vi "30-20-10-2.vi"() -> ()   [LabVIEW 2025]
uses:
  <vilib>/Platform/TimedLoop/XDataNode/timing_clust.ctl
  <vilib>/Platform/TimedLoop/XDataNode/nitl_modes.ctl
  <vilib>/Platform/TimedLoop/XDataNode/wakeup.ctl
  <vilib>/rvi/Emulation/niFpgaSctlEmulationGetInTimedLoop.vi
  <vilib>/rvi/Emulation/niFpgaEmulationReportErrorSimple.vi
  <vilib>/rvi/Emulation/niFpgaGetClockAttributes.vi
  <vilib>/rvi/Emulation/niFpgaCriticalErrorInLSC.vi
  <vilib>/rvi/linearAlgebra/MatrixMultiply/simVIs/SubVI/nifxpla_MatrixMultiply_SimMatrixSizes.vi
  <vilib>/rvi/linearAlgebra/MatrixMultiply/simVIs/SubVI/nifxpla_MatrixMultiply_Sim4WireAdapterVector.vi
  <vilib>/rvi/linearAlgebra/MatrixMultiply/simVIs/SubVI/nifxpla_MatrixMultiply_SimFrameHandShake.vi
  <vilib>/rvi/linearAlgebra/MatrixMultiply/simVIs/SubVI/nifxpla_MatrixMultiply_SimEndlessCounter.vi
  <vilib>/rvi/linearAlgebra/MatrixMultiply/simVIs/SubVI/nifxpla_MatrixMultiply_SimVectorDataBuffer.vi
  <vilib>/rvi/ClientSDK/Core/DevComputerLib/Private/Multiply(dfxp64).vi
  <vilib>/rvi/ClientSDK/Core/DevComputerLib/Private/Dfxp128ToDfxp256.vi
  <vilib>/rvi/ClientSDK/Core/DevComputerLib/Private/Add(dfxp256).vi
  <vilib>/rvi/ClientSDK/Core/DevComputerLib/Private/Subtract(dfxp256).vi
  <vilib>/rvi/ClientSDK/Core/DevComputerLib/Private/ToDfxp64(dfxp256).vi
  <vilib>/platform/TimedLoop/XDataNode/XDataNode.xnode
  <vilib>/rvi/linearAlgebra/MatrixMultiply/XNode/nifxpla_MatrixMultiply.xnode
  <vilib>/rvi/linearAlgebra/MatrixMultiply/simVIs/nifxpla_MatrixMultiply_SimTemplateEinEout.vi
  <vilib>/rvi/linearAlgebra/MatrixMultiply/simVIs/nifxpla_MatrixMultiply_SimTemplateEinVout.vi
  <vilib>/rvi/linearAlgebra/MatrixMultiply/simVIs/nifxpla_MatrixMultiply_SimTemplateVinEout.vi
  <vilib>/rvi/linearAlgebra/MatrixMultiply/simVIs/nifxpla_MatrixMultiply_SimTemplateVinVout.vi
  <vilib>/Platform/TimedLoop/XDataNode/XDNodeRunTimeDep.lvlib
panel:
  out "Latency":u32
  out "Cycle Count 3":i32
  out "C3":fxp<+/-,32,16>[](array[numeric])
  out "C3+B":fxp<+/-,33,17>[](array[numeric])
  out "Cycle Count 2":i32
  out "C2":fxp<+/-,32,16>[](array[numeric])
  out "C2+B":fxp<+/-,33,17>[](array[numeric])
  out "Cycle Count":i32
  out "C1":fxp<+/-,32,16>[](array[numeric])
  out "C1+B":fxp<+/-,33,17>[](array[numeric])
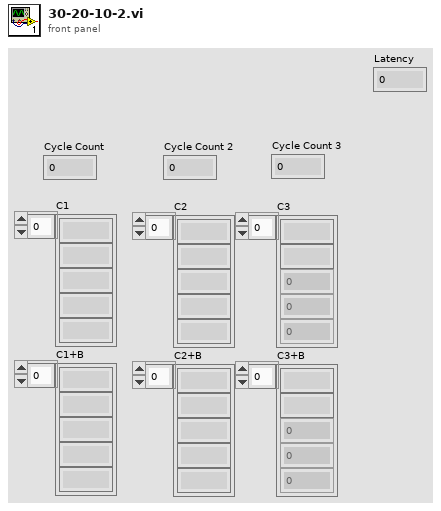
[diagram p1: front panel]
types:
  T1 = typedef "XDNodeRunTimeDep.lvlib/timing_clust.ctl" = cluster{"Expected End [f-1]":u64, "Actual End [f-1]":u64, "Finished Late? [f-1]":bool, "Expected End [i-1]":u64, "Actual End [i-1]":u64, "Finished Late? [i-1]":bool, "Expected Start [i]":u64, "Actual Start [i]":u64, "Expected Start [f]":u64, "Actual Start [f]":u64, "Source Name":string, "Structure Name":string, "Period":i64, "Deadline":i64, "Offset":i64, "Start":i64, "Priority":i32, "Timeout":i32, "Mode":T2, "Wakeup Reason":T3, "Error":errorcluster, "Source Type":string, "Secondary Source Type":string, "Global End Time":u64, "Global Start Time":u64, "Frame Duration":u64, "Iteration Duration":u64, "Assigned CPU":i32, "I/O Scan Engine Mode":u32}
  T2 = typedef "XDNodeRunTimeDep.lvlib/nitl_modes.ctl" = enum32{"No Change", "Process missed periods, maintain original phase", "Discard missed periods, maintain original phase", "Process missed periods, ignore original phase", "Discard missed periods, ignore original phase"}
  T3 = typedef "XDNodeRunTimeDep.lvlib/wakeup.ctl" = enum32{"Normal", "Aborted", "Asynchronous wakeup", "Timing source error", "Timed loop error", "Timeout"}
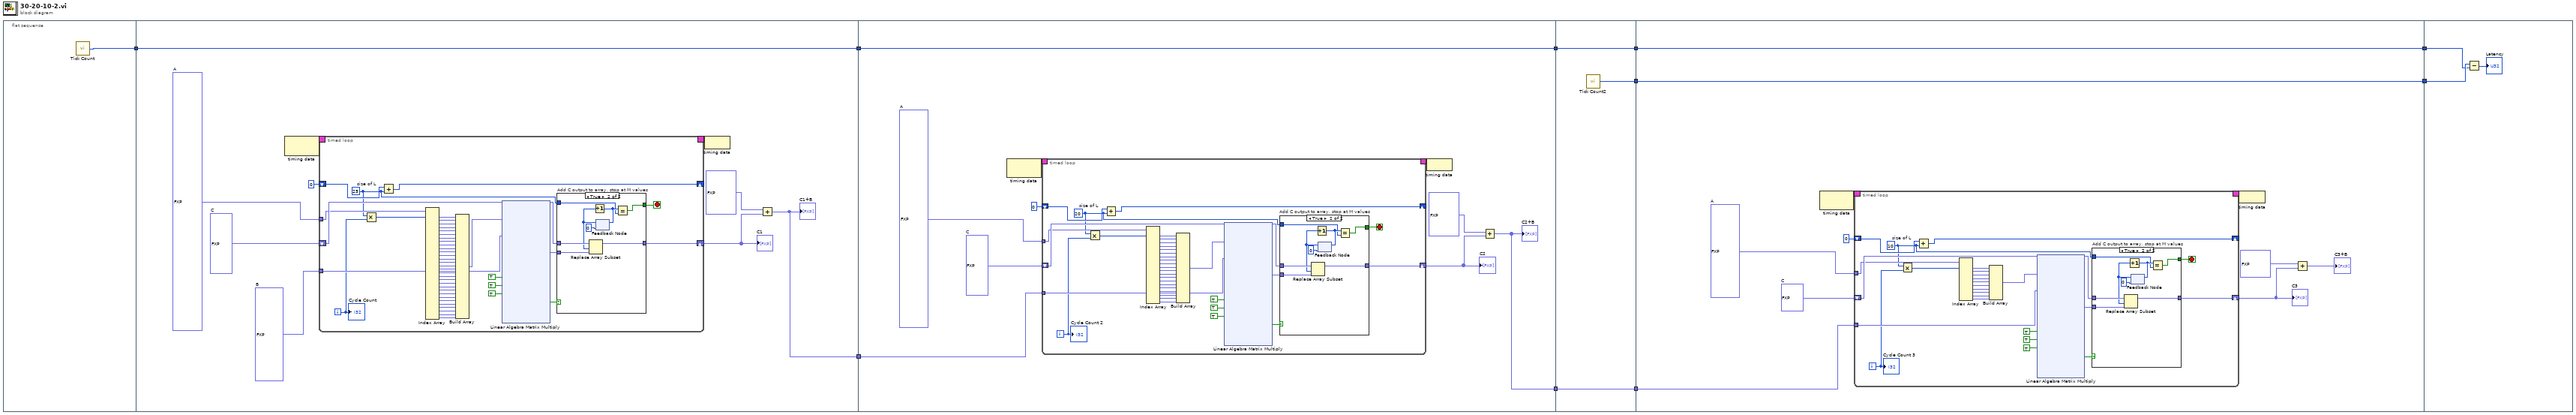
[diagram p0: block diagram]
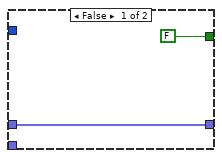
[diagram p2: hidden frame]
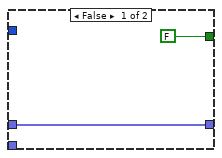
[diagram p3: hidden frame]
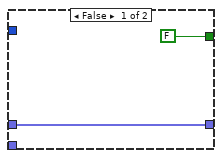
[diagram p4: hidden frame]
diagram:
  n1 = flat-sequence {
    tunnel: [w11] -> w10
    tunnel: [w13] -> w9
    tunnel: [w12] -> w8
    tunnel: w10 -> [w12]
    tunnel: w9 -> [w84]
    tunnel: [w83] -> w7
    tunnel: w8 -> [w82]
    tunnel: [w82] -> w6
    tunnel: w7 -> [w144]
    tunnel: [w144] -> w5
    tunnel: w6 -> [w143]
    tunnel: [w143] -> w4
    tunnel: [w142] -> w3
    tunnel: w5 -> [w147]
    tunnel: w4 -> [w146]
    tunnel: [w146] -> w2
    tunnel: [w145] -> w1
    tunnel: w3 -> [w145]
    tunnel: w2 -> [w197]
    tunnel: w1 -> [w198]
    frame #0 {
      n2 = call "Tick Count"() -> ("Tick Count(Ticks)"=w11:u32)
    }
    frame #1 {
      w17 = fxp<+/-,32,16>[] [0.0, 0.0, 0.0, 0.0, 0.0, 0.0, 0.0, 0.0, 0.0, 0.0, 0.0, 0.0, 0.0, 0.0, 0.0, 0.0, 0.0, 0.0, 0.0, 0.0, 0.0, 0.0, 0.0, 0.0, 0.0, 0.0, 0.0, 0.0, 0.0, 0.0, 0.0, 0.0, 0.0, 0.0, 0.0, 0.0, 0.0, 0.0, 0.0, 0.0, 0.0, 0.0, 0.0, 0.0, 0.0, 0.0, 0.0, 0.0, 0.0, 0.0, 0.0, 0.0, 0.0, 0.0, 0.0, 0.0, 0.0, 0.0, 0.0, 0.0, 0.0, 0.0, 0.0, 0.0, 0.0, 0.0, 0.0, 0.0, 0.0, 0.0, 0.0, 0.0, 0.0, 0.0, 0.0, 0.0, 0.0, 0.0, 0.0, 0.0, 0.0, 0.0, 0.0, 0.0, 0.0, 0.0, 0.0, 0.0, 0.0, 0.0, 0.0, 0.0, 0.0, 0.0, 0.0, 0.0, 0.0, 0.0, 0.0, 0.0, 0.0, 0.0, 0.0, 0.0, 0.0, 0.0, 0.0, 0.0, 0.0, 0.0, 0.0, 0.0, 0.0, 0.0, 0.0, 0.0, 0.0, 0.0, 0.0, 0.0, 0.0, 0.0, 0.0, 0.0, 0.0, 0.0, 0.0, 0.0, 0.0, 0.0, 0.0, 0.0, 0.0, 0.0, 0.0, 0.0, 0.0, 0.0, 0.0, 0.0, 0.0, 0.0, 0.0, 0.0, 0.0, 0.0, 0.0, 0.0, 0.0, 0.0, 0.0, 0.0, 0.0, 0.0, 0.0, 0.0, 0.0, 0.0, 0.0, 0.0, 0.0, 0.0, 0.0, 0.0, 0.0, 0.0, 0.0, 0.0, 0.0, 0.0, 0.0, 0.0, 0.0, 0.0, 0.0, 0.0, 0.0, 0.0, 0.0, 0.0, 0.0, 0.0, 0.0, 0.0, 0.0, 0.0, 0.0, 0.0, 0.0, 0.0, 0.0, 0.0, 0.0, 0.0, 0.0, 0.0, 0.0, 0.0, 0.0, 0.0, 0.0, 0.0, 0.0, 0.0, 0.0, 0.0, 0.0, 0.0, 0.0, 0.0, 0.0, 0.0, 0.0, 0.0, 0.0, 0.0, 0.0, 0.0, 0.0, 0.0, 0.0, 0.0, 0.0, 0.0, 0.0, 0.0, 0.0, 0.0, 0.0, 0.0, 0.0, 0.0, 0.0, 0.0, 0.0, 0.0, 0.0, 0.0, 0.0, 0.0, 0.0, 0.0, 0.0, 0.0, 0.0, 0.0, 0.0, 0.0, 0.0, 0.0, 0.0, 0.0, 0.0, 0.0, 0.0, 0.0, 0.0, 0.0, 0.0, 0.0, 0.0, 0.0, 0.0, 0.0, 0.0, 0.0, 0.0, 0.0, 0.0, 0.0, 0.0, 0.0, 0.0, 0.0, 0.0, 0.0, 0.0, 0.0, 0.0, 0.0, 0.0, 0.0, 0.0, 0.0, 0.0, 0.0, 0.0, 0.0, 0.0, 0.0, 0.0, 0.0, 0.0, 0.0, 0.0, 0.0, 0.0, 0.0, 0.0, 0.0, 0.0, 0.0, 0.0, 0.0, 0.0, 0.0, 0.0, 0.0, 0.0, 0.0, 0.0, 0.0, 0.0, 0.0, 0.0, 0.0, 0.0, 0.0, 0.0, 0.0, 0.0, 0.0, 0.0, 0.0, 0.0, 0.0, 0.0, 0.0, 0.0, 0.0, 0.0, 0.0, 0.0, 0.0, 0.0, 0.0, 0.0, 0.0, 0.0, 0.0, 0.0, 0.0, 0.0, 0.0, 0.0, 0.0, 0.0, 0.0, 0.0, 0.0, 0.0, 0.0, 0.0, 0.0, 0.0, 0.0, 0.0, 0.0, 0.0, 0.0, 0.0, 0.0, 0.0, 0.0, 0.0, 0.0, 0.0, 0.0, 0.0, 0.0, 0.0, 0.0, 0.0, 0.0, 0.0, 0.0, 0.0, 0.0, 0.0, 0.0, 0.0, 0.0, 0.0, 0.0, 0.0, 0.0, 0.0, 0.0, 0.0, 0.0, 0.0, 0.0, 0.0, 0.0, 0.0, 0.0, 0.0, 0.0, 0.0, 0.0, 0.0, 0.0, 0.0, 0.0, 0.0, 0.0, 0.0, 0.0, 0.0, 0.0, 0.0, 0.0, 0.0, 0.0, 0.0, 0.0, 0.0, 0.0, 0.0, 0.0, 0.0, 0.0, 0.0, 0.0, 0.0, 0.0, 0.0, 0.0, 0.0, 0.0, 0.0, 0.0, 0.0, 0.0, 0.0, 0.0, 0.0, 0.0, 0.0, 0.0, 0.0, 0.0, 0.0, 0.0, 0.0, 0.0, 0.0, 0.0, 0.0, 0.0, 0.0, 0.0, 0.0, 0.0, 0.0, 0.0, 0.0, 0.0, 0.0, 0.0, 0.0, 0.0, 0.0, 0.0, 0.0, 0.0, 0.0, 0.0, 0.0, 0.0, 0.0, 0.0, 0.0, 0.0, 0.0, 0.0, 0.0, 0.0, 0.0, 0.0, 0.0, 0.0, 0.0, 0.0, 0.0, 0.0, 0.0, 0.0, 0.0, 0.0, 0.0, 0.0, 0.0, 0.0, 0.0, 0.0, 0.0, 0.0, 0.0, 0.0, 0.0, 0.0, 0.0, 0.0, 0.0, 0.0, 0.0, 0.0, 0.0, 0.0, 0.0, 0.0, 0.0, 0.0, 0.0, 0.0, 0.0, 0.0, 0.0, 0.0, 0.0, 0.0, 0.0, 0.0, 0.0, 0.0, 0.0, 0.0, 0.0, 0.0, 0.0, 0.0, 0.0, 0.0, 0.0, 0.0, 0.0, 0.0, 0.0, 0.0, 0.0, 0.0, 0.0, 0.0, 0.0, 0.0, 0.0, 0.0, 0.0, 0.0, 0.0, 0.0, 0.0, 0.0, 0.0, 0.0, 0.0, 0.0, 0.0, 0.0, 0.0, 0.0, 0.0, 0.0, 0.0, 0.0, 0.0, 0.0, 0.0, 0.0, 0.0, 0.0, 0.0, 0.0, 0.0, 0.0, 0.0, 0.0, 0.0, 0.0, 0.0, 0.0, 0.0, 0.0, 0.0, 0.0, 0.0, 0.0, 0.0, 0.0, 0.0, 0.0, 0.0, 0.0, 0.0, 0.0, 0.0, 0.0, 0.0, 0.0]  # A
      w18 = fxp<+/-,32,16>[] [0.0, 0.0, 0.0, 0.0, 0.0, 0.0, 0.0, 0.0, 0.0, 0.0, 0.0, 0.0, 0.0, 0.0, 0.0, 0.0, 0.0, 0.0, 0.0, 0.0, 0.0, 0.0, 0.0, 0.0, 0.0, 0.0, 0.0, 0.0, 0.0, 0.0]  # B
      w19 = fxp<+/-,32,16>[] [0.0, 0.0, 0.0, 0.0, 0.0, 0.0, 0.0, 0.0, 0.0, 0.0, 0.0, 0.0, 0.0, 0.0, 0.0, 0.0, 0.0, 0.0, 0.0, 0.0]  # C
      n3 = node-c288() -> (w21:T1)  [unwired: 1 in]
      n4 = timed-loop {
        timing: w21 -> [_]
        timing-out: [_] -> w20
        shift-right: [w66] -> w15
        shift-left: w19 -> [w65]
        tunnel: w18 -> [w62]
        tunnel: w17 -> [w45]
        shift-right: [w58] -> _
        shift-left: 0 ("length") -> [w59]
        i -> [w44]
        stop <- w64 stop-if-true
        w43 = 25  # size of L
        n5 = Multiply(x=w43, y=w44) -> (x*y=w56:i32)
        n6 = Add(x=w59, y=w43) -> (x+y=w58:i32)
        n7 = Index Array(array=w45, index #1=w56) -> (element #1=w55:fxp<+/-,32,16>, element #2=w54:fxp<+/-,32,16>, element #3=w53:fxp<+/-,32,16>, element #4=w52:fxp<+/-,32,16>, element #5=w51:fxp<+/-,32,16>, element #6=w50:fxp<+/-,32,16>, element #7=w49:fxp<+/-,32,16>, element #8=w48:fxp<+/-,32,16>, element #9=w47:fxp<+/-,32,16>, element #10=w46:fxp<+/-,32,16>, element #11=w41:fxp<+/-,32,16>, element #12=w40:fxp<+/-,32,16>, element #13=w39:fxp<+/-,32,16>, element #14=w38:fxp<+/-,32,16>, element #15=w37:fxp<+/-,32,16>, element #16=w36:fxp<+/-,32,16>, element #17=w35:fxp<+/-,32,16>, element #18=w34:fxp<+/-,32,16>, element #19=w33:fxp<+/-,32,16>, element #20=w32:fxp<+/-,32,16>, element #21=w31:fxp<+/-,32,16>, element #22=w30:fxp<+/-,32,16>, element #23=w29:fxp<+/-,32,16>, element #24=w28:fxp<+/-,32,16>, element #25=w27:fxp<+/-,32,16>, element #26=w26:fxp<+/-,32,16>, element #27=w25:fxp<+/-,32,16>, element #28=w24:fxp<+/-,32,16>, element #29=w23:fxp<+/-,32,16>, element #30=w22:fxp<+/-,32,16>)  [unwired: 29 in]
        n8 = Build Array(w55, w54, w53, w52, w51, w50, w49, w48, w47, w46, w41, w40, w39, w38, w37, w36, w35, w34, w33, w32, w31, w30, w29, w28, w27, w26, w25, w24, w23, w22) -> (w42:fxp<+/-,32,16>[])
        n9 = xnode ("Linear Algebra Matrix Multiply")("ar"=w42, "br"=w62, "a valid"=TRUE, "b valid"=TRUE, "ready for output (T)"=TRUE) -> ("cr"=w61:fxp<+/-,64,37>[], "output valid"=w57:bool)  [unwired: 2 in, 4 out]
        n10 = case "Add C output to array, stop at M values" shown="True" w57 {
          tunnel: w61 -> [_ w73]
          tunnel: [w69 w76] -> w66
          tunnel: w65 -> [w69 w77]
          tunnel: [FALSE w74] -> w64
          tunnel: w43 -> [_ w70]
          frame False {
          }
          frame True {
            n11 = feedback #1(0 ("x")) -> (w72:i32)
            n12 = Replace Array Subset(array=w77, new element=w73, index=w72) -> (w76:fxp<+/-,32,16>[])
            n13 = Increment(x=w72) -> (x+1=w71:i32)
            n14 = feedback-in #1(w71) -> ()
            n15 = Equal?(x=w71, y=w70) -> (x = y?=w74:bool)
          }
        }
        "Cycle Count" <- w44
      }
      "C1" <- w15
      n16 = node-c288(w20) -> ()
      n17 = Add(x=fxp<+/-,32,16>[] [0.5, 0.5, 0.5, 0.5, 0.5, 0.0, 0.0, 0.0, 0.0, 0.0, 0.0, 0.0, 0.0, 0.0, 0.0, 0.0, 0.0, 0.0, 0.0, 0.0], y=w15) -> (x+y=w13:fxp<+/-,33,17>[])
      "C1+B" <- w13
    }
    frame #2 {
      w88 = fxp<+/-,32,16>[] [0.0, 0.0, 0.0, 0.0, 0.0, 0.0, 0.0, 0.0, 0.0, 0.0, 0.0, 0.0, 0.0, 0.0, 0.0, 0.0, 0.0, 0.0, 0.0, 0.0, 0.0, 0.0, 0.0, 0.0, 0.0, 0.0, 0.0, 0.0, 0.0, 0.0, 0.0, 0.0, 0.0, 0.0, 0.0, 0.0, 0.0, 0.0, 0.0, 0.0, 0.0, 0.0, 0.0, 0.0, 0.0, 0.0, 0.0, 0.0, 0.0, 0.0, 0.0, 0.0, 0.0, 0.0, 0.0, 0.0, 0.0, 0.0, 0.0, 0.0, 0.0, 0.0, 0.0, 0.0, 0.0, 0.0, 0.0, 0.0, 0.0, 0.0, 0.0, 0.0, 0.0, 0.0, 0.0, 0.0, 0.0, 0.0, 0.0, 0.0, 0.0, 0.0, 0.0, 0.0, 0.0, 0.0, 0.0, 0.0, 0.0, 0.0, 0.0, 0.0, 0.0, 0.0, 0.0, 0.0, 0.0, 0.0, 0.0, 0.0, 0.0, 0.0, 0.0, 0.0, 0.0, 0.0, 0.0, 0.0, 0.0, 0.0, 0.0, 0.0, 0.0, 0.0, 0.0, 0.0, 0.0, 0.0, 0.0, 0.0, 0.0, 0.0, 0.0, 0.0, 0.0, 0.0, 0.0, 0.0, 0.0, 0.0, 0.0, 0.0, 0.0, 0.0, 0.0, 0.0, 0.0, 0.0, 0.0, 0.0, 0.0, 0.0, 0.0, 0.0, 0.0, 0.0, 0.0, 0.0, 0.0, 0.0, 0.0, 0.0, 0.0, 0.0, 0.0, 0.0, 0.0, 0.0, 0.0, 0.0, 0.0, 0.0, 0.0, 0.0, 0.0, 0.0, 0.0, 0.0, 0.0, 0.0, 0.0, 0.0, 0.0, 0.0, 0.0, 0.0, 0.0, 0.0, 0.0, 0.0, 0.0, 0.0, 0.0, 0.0, 0.0, 0.0, 0.0, 0.0, 0.0, 0.0, 0.0, 0.0, 0.0, 0.0, 0.0, 0.0, 0.0, 0.0, 0.0, 0.0]  # A
      w89 = fxp<+/-,32,16>[] [0.0, 0.0, 0.0, 0.0, 0.0, 0.0, 0.0, 0.0, 0.0, 0.0]  # C
      n18 = node-c288() -> (w91:T1)  [unwired: 1 in]
      n19 = timed-loop {
        timing: w91 -> [_]
        timing-out: [_] -> w90
        shift-right: [w126] -> w86
        shift-left: w89 -> [w125]
        tunnel: w84 -> [w122]
        tunnel: w88 -> [w110]
        shift-right: [w118] -> _
        shift-left: 0 ("length") -> [w119]
        i -> [w109]
        stop <- w124 stop-if-true
        w108 = 20  # size of L
        n20 = Multiply(x=w108, y=w109) -> (x*y=w116:i32)
        n21 = Add(x=w119, y=w108) -> (x+y=w118:i32)
        n22 = Index Array(array=w110, index #1=w116) -> (element #1=w115:fxp<+/-,32,16>, element #2=w114:fxp<+/-,32,16>, element #3=w113:fxp<+/-,32,16>, element #4=w112:fxp<+/-,32,16>, element #5=w111:fxp<+/-,32,16>, element #6=w106:fxp<+/-,32,16>, element #7=w105:fxp<+/-,32,16>, element #8=w104:fxp<+/-,32,16>, element #9=w103:fxp<+/-,32,16>, element #10=w102:fxp<+/-,32,16>, element #11=w101:fxp<+/-,32,16>, element #12=w100:fxp<+/-,32,16>, element #13=w99:fxp<+/-,32,16>, element #14=w98:fxp<+/-,32,16>, element #15=w97:fxp<+/-,32,16>, element #16=w96:fxp<+/-,32,16>, element #17=w95:fxp<+/-,32,16>, element #18=w94:fxp<+/-,32,16>, element #19=w93:fxp<+/-,32,16>, element #20=w92:fxp<+/-,32,16>)  [unwired: 19 in]
        n23 = Build Array(w115, w114, w113, w112, w111, w106, w105, w104, w103, w102, w101, w100, w99, w98, w97, w96, w95, w94, w93, w92) -> (w107:fxp<+/-,32,16>[])
        n24 = xnode ("Linear Algebra Matrix Multiply")("ar"=w107, "br"=w122, "a valid"=TRUE, "b valid"=TRUE, "ready for output (T)"=TRUE) -> ("cr"=w121:fxp<+/-,64,38>[], "output valid"=w117:bool)  [unwired: 2 in, 4 out]
        n25 = case "Add C output to array, stop at M values" shown="True" w117 {
          tunnel: w121 -> [_ w133]
          tunnel: [w129 w136] -> w126
          tunnel: w125 -> [w129 w137]
          tunnel: [FALSE w134] -> w124
          tunnel: w108 -> [_ w130]
          frame False {
          }
          frame True {
            n26 = feedback #2(0 ("x")) -> (w132:i32)
            n27 = Replace Array Subset(array=w137, new element=w133, index=w132) -> (w136:fxp<+/-,32,16>[])
            n28 = Increment(x=w132) -> (x+1=w131:i32)
            n29 = feedback-in #2(w131) -> ()
            n30 = Equal?(x=w131, y=w130) -> (x = y?=w134:bool)
          }
        }
        "Cycle Count 2" <- w109
      }
      "C2" <- w86
      n31 = node-c288(w90) -> ()
      n32 = Add(x=fxp<+/-,32,16>[] [0.5, 0.5, 0.5, 0.5, 0.5, 0.0, 0.0, 0.0, 0.0, 0.0], y=w86) -> (x+y=w83:fxp<+/-,33,17>[])
      "C2+B" <- w83
    }
    frame #3 {
      n33 = call "Tick Count2"() -> ("Tick Count(Ticks)"=w142:u32)
    }
    frame #4 {
      w152 = fxp<+/-,32,16>[] [0.0, 0.0, 0.0, 0.0, 0.0, 0.0, 0.0, 0.0, 0.0, 0.0, 0.0, 0.0, 0.0, 0.0, 0.0, 0.0, 0.0, 0.0, 0.0, 0.0]  # A
      w153 = fxp<+/-,32,16>[] [0.0, 0.0]  # C
      n34 = node-c288() -> (w155:T1)  [unwired: 1 in]
      n35 = timed-loop {
        timing: w155 -> [_]
        timing-out: [_] -> w154
        shift-right: [w180] -> w150
        shift-left: w153 -> [w179]
        tunnel: w147 -> [w176]
        tunnel: w152 -> [w164]
        shift-right: [w172] -> _
        shift-left: 0 ("length") -> [w173]
        i -> [w163]
        stop <- w178 stop-if-true
        w162 = 10  # size of L
        n36 = Multiply(x=w162, y=w163) -> (x*y=w170:i32)
        n37 = Add(x=w173, y=w162) -> (x+y=w172:i32)
        n38 = Index Array(array=w164, index #1=w170) -> (element #1=w169:fxp<+/-,32,16>, element #2=w168:fxp<+/-,32,16>, element #3=w167:fxp<+/-,32,16>, element #4=w166:fxp<+/-,32,16>, element #5=w165:fxp<+/-,32,16>, element #6=w159:fxp<+/-,32,16>, element #7=w160:fxp<+/-,32,16>, element #8=w158:fxp<+/-,32,16>, element #9=w157:fxp<+/-,32,16>, element #10=w156:fxp<+/-,32,16>)  [unwired: 9 in]
        n39 = Build Array(w169, w168, w167, w166, w165, w159, w160, w158, w157, w156) -> (w161:fxp<+/-,32,16>[])
        n40 = xnode ("Linear Algebra Matrix Multiply")("ar"=w161, "br"=w176, "a valid"=TRUE, "b valid"=TRUE, "ready for output (T)"=TRUE) -> ("cr"=w175:fxp<+/-,64,37>[], "output valid"=w171:bool)  [unwired: 2 in, 4 out]
        n41 = case "Add C output to array, stop at M values" shown="True" w171 {
          tunnel: w175 -> [_ w187]
          tunnel: [w183 w190] -> w180
          tunnel: w179 -> [w183 w191]
          tunnel: [FALSE w188] -> w178
          tunnel: w162 -> [_ w184]
          frame False {
          }
          frame True {
            n42 = feedback #3(0 ("x")) -> (w186:i32)
            n43 = Replace Array Subset(array=w191, new element=w187, index=w186) -> (w190:fxp<+/-,32,16>[])
            n44 = Increment(x=w186) -> (x+1=w185:i32)
            n45 = feedback-in #3(w185) -> ()
            n46 = Equal?(x=w185, y=w184) -> (x = y?=w188:bool)
          }
        }
        "Cycle Count 3" <- w163
      }
      "C3" <- w150
      n47 = node-c288(w154) -> ()
      n48 = Add(x=fxp<+/-,32,16>[] [0.5, 0.5], y=w150) -> (x+y=→"C3+B":fxp<+/-,33,17>[])
    }
    frame #5 {
      n49 = Subtract(x=w198, y=w197) -> (x-y=→"Latency":u32)
    }
  }
